vi "BuildCTRL2Word.vi"(11 "NewVal":T1) -> (3 "string":string)   [LabVIEW 2020, in "CTI-Peripheral.lvlib" / "Adafruit NAU7802 24bit Strain Gauge.lvclass"]
uses:
  Adafruit NAU7802 24bit Strain Gauge.lvclass
  NAU7802DataRate.ctl
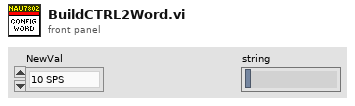
[diagram p1: front panel]
types:
  T1 = typedef "CTI-Peripheral.lvlib/Adafruit NAU7802 24bit Strain Gauge.lvclass/NAU7802DataRate.ctl" = enum16{"10 SPS", "20 SPS", "40 SPS", "80 SPS", "320 SPS"}
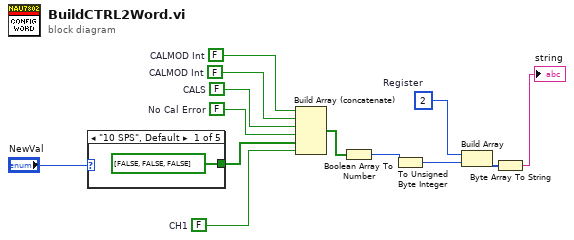
[diagram p0: block diagram]
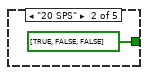
[diagram p2: hidden frame]
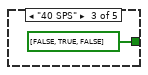
[diagram p3: hidden frame]
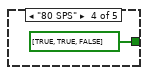
[diagram p4: hidden frame]
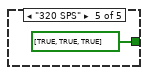
[diagram p5: hidden frame]
diagram:
  w1 = FALSE  # CALMOD Int
  w2 = FALSE  # CALMOD Int
  w3 = FALSE  # CALS
  w4 = FALSE  # No Cal Error
  w5 = FALSE  # CH1
  w10 = u8 2  # Register
  n1 = case shown="\"10 SPS\", Default" "NewVal" {
    tunnel: [bool[] [FALSE, FALSE, FALSE] bool[] [TRUE, FALSE, FALSE] bool[] [FALSE, TRUE, FALSE] bool[] [TRUE, TRUE, FALSE] bool[] [TRUE, TRUE, TRUE]] -> w11
    frame "10 SPS", Default {
    }
    frame "20 SPS" {
    }
    frame "40 SPS" {
    }
    frame "80 SPS" {
    }
    frame "320 SPS" {
    }
  }
  n2 = Build Array (concatenate)(w2, w1, w3, w4, w11, w5) -> (w9:bool[])
  n3 = Boolean Array To Number(Boolean array=w9) -> (number=w8:u32)
  n4 = To Unsigned Byte Integer(number=w8) -> (unsigned 8bit integer=w7:u8)
  n5 = Build Array(w10, w7) -> (w12:u8[])
  n6 = Byte Array To String(unsigned byte array=w12) -> (string=→"string":string)
